vi "Configure Control AI RJC.vi"(0 "VISA resource name":refnum<visa-resource-name>, 1 "Unit No. (0)":i32 min=0 max=6, 4 "Module No.(0)":i32 min=0 max=9, 5 "AI No.(1)":i32=1 min=1 max=2, 7 "error in (no error)":errorcluster, 8 "Temperature":dbl=2.0 min=0.0 max=2.0 format="%.1f", 9 "Mode(0:Internal)":i32 min=0 max=1) -> (20 "VISA resource name out":refnum<visa-resource-name>, 21 "AI No.":i32, 24 "Unit No.":i32, 25 "Module No.":i32, 27 "error out":errorcluster)   [LabVIEW 2020, in "Yokogawa GX Series.lvlib"]
doc: "Set the reference junction compensation temperature of AI of PID module.\n\nCommand: SCtrlRjc"
uses:
  <instrlib>/Yokogawa GX Series/Yokogawa GX Series.lvlib
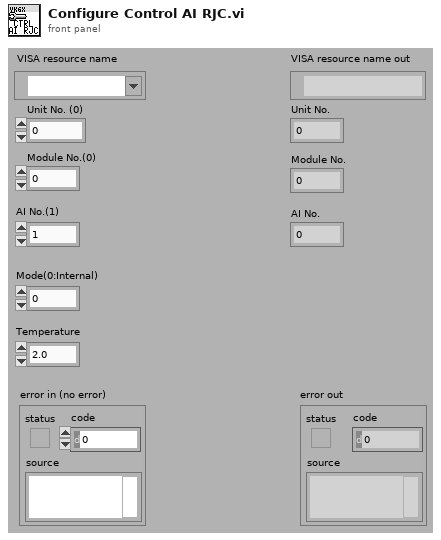
[diagram p1: front panel]
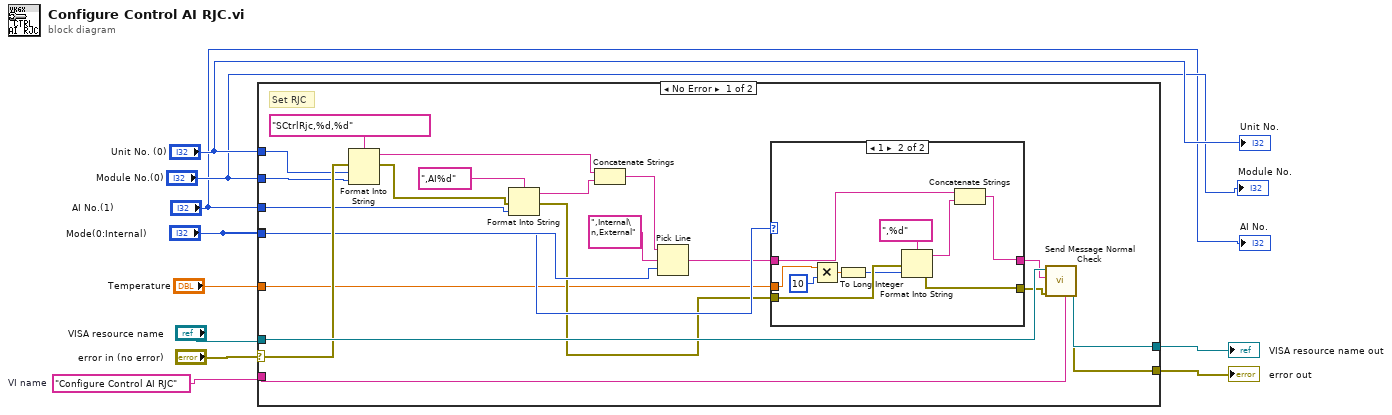
[diagram p0: block diagram]
diagram:
  w6 = "Configure Control AI RJC"  # VI name
  n1 = case shown="No Error" "error in (no error)" {
    selector: "error in (no error)" -> [w28 w45]
    tunnel: [w32 w46] -> w10
    tunnel: [w31 w45] -> w9
    tunnel: "VISA resource name" -> [w30 w46]
    tunnel: w6 -> [w27 _]
    tunnel: "Unit No. (0)" -> [w24 _]
    tunnel: "Module No.(0)" -> [w23 _]
    tunnel: "Mode(0:Internal)" -> [w25 _]
    tunnel: "AI No.(1)" -> [w21 _]
    tunnel: "Mode(0:Internal)" -> [w16 _]
    tunnel: "Temperature" -> [w11 _]
    frame No Error {
      # "Set RJC"
      n2 = Format Into String(format string="SCtrlRjc,%d,%d", error in=w28, w24, w23) -> (resulting string=w19:string, error out=w20:errorcluster)  [unwired: 1 in]
      n3 = Format Into String(format string=",AI%d", error in=w20, w21) -> (resulting string=w18:string, error out=w13:errorcluster)  [unwired: 1 in]
      n4 = Concatenate Strings(w19, w18) -> (w17:string)
      n5 = Pick Line(string ("")=w17, multi-line string=",Internal\n,External", line index=w25) -> (output string=w15:string)
      n6 = case shown="1" w16 {
        tunnel: w15 -> [w34 w41]
        tunnel: [w34 w39] -> w14
        tunnel: w13 -> [w33 w43]
        tunnel: [w33 w42] -> w12
        tunnel: w11 -> [_ w38]
        frame 0, Default {
        }
        frame 1 {
          n7 = Multiply(x=w38, y=10) -> (x*y=w36:dbl)
          n8 = To Long Integer(number=w36) -> (32bit integer=w35:i32)
          n9 = Format Into String(format string=",%d", error in=w43, w35) -> (resulting string=w40:string, error out=w42:errorcluster)  [unwired: 1 in]
          n10 = Concatenate Strings(w41, w40) -> (w39:string)
        }
      }
      n11 = call <instrlib>:"Send Message Normal Check.vi"("Source (\"\")"=w27, "error in (no error)"=w12, "Send Message (\"\")"=w14, "VISA resource name"=w30) -> ("error out"=w31:errorcluster, "VISA resource name out"=w32:refnum<visa-resource-name>)  [unwired: 2 in, 4 out]
    }
    frame Error {
    }
  }
  "error out" <- w9
  "VISA resource name out" <- w10
  "Unit No." <- "Unit No. (0)"
  "Module No." <- "Module No.(0)"
  "AI No." <- "AI No.(1)"
